vi "Distancias_ejes_convoy_baja_velocidad.vi"(3 "Radios ruedas":dbl[](array[numeric]), 4 "Series_flota1":string[](array[string]), 5 "Ejes_UT":i32[](array[numeric]), 6 "Puntos medios de las ventanas":dbl[][](array[numeric]), 7 "Series_flota":string[](array[string])) -> (0 "Radios_por_ejes":dbl[](array[numeric]), 1 "Distancias_entre_ejes_convoy":dbl[](array[numeric]))   [LabVIEW 2015]
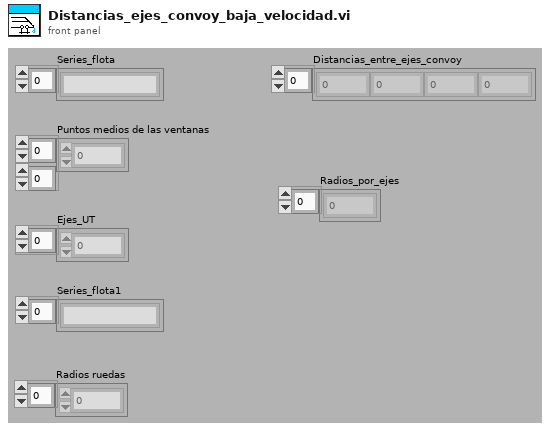
[diagram p1: front panel]
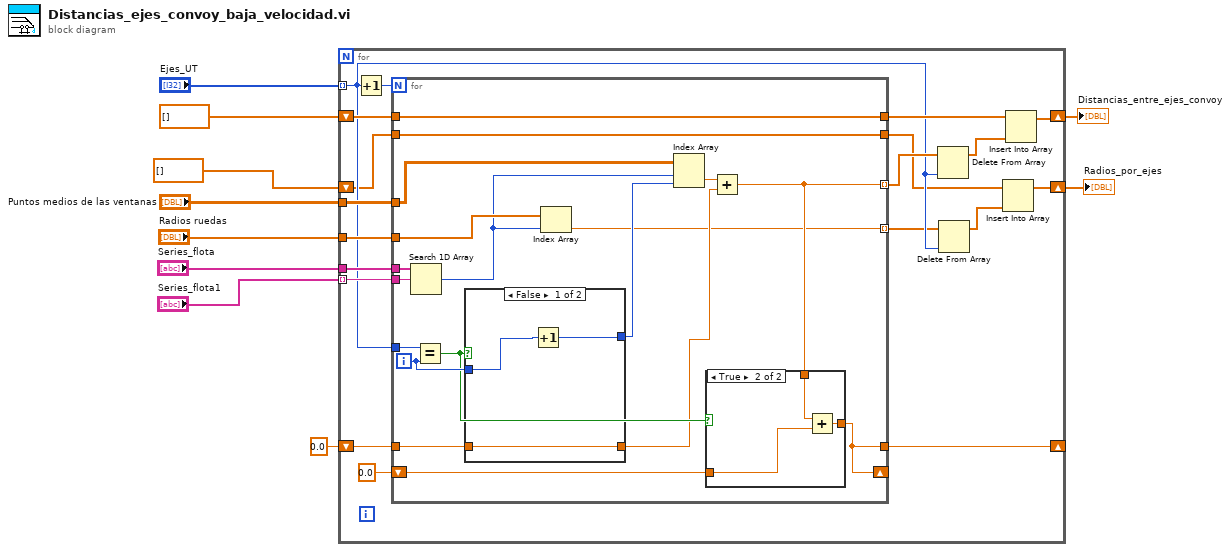
[diagram p0: block diagram]
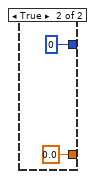
[diagram p3: hidden frame]
diagram:
  n1 = for {
    tunnel: "Puntos medios de las ventanas" -> [w29]
    tunnel: "Ejes_UT" -> [w16] mode=indexing
    tunnel: "Series_flota" -> [w27]
    tunnel: "Series_flota1" -> [w26] mode=indexing
    shift-right: [w23] -> w8
    shift-left: dbl[] [] -> [w25]
    shift-right: [w18] -> _
    shift-left: 0.0 -> [w19]
    tunnel: "Radios ruedas" -> [w17]
    shift-right: [w11] -> w1
    shift-left: dbl[] [] -> [w13]
    n2 = Increment(x=w16) -> (x+1=w28:i32)
    n3 = for {
      N: w28 -> [_]
      tunnel: w29 -> [w42]
      tunnel: w16 -> [w45]
      tunnel: w27 -> [w44]
      tunnel: w26 -> [w43]
      tunnel: [w39] -> w22 mode=indexing
      tunnel: w25 -> [w41]
      tunnel: [w41] -> w24
      shift-right: [w37] -> _
      shift-left: 0.0 -> [w40]
      tunnel: w19 -> [w35]
      tunnel: [w37] -> w18
      tunnel: w17 -> [w33]
      tunnel: [w31] -> w15 mode=indexing
      tunnel: [w30] -> w12
      tunnel: w13 -> [w30]
      i -> [w47]
      n4 = Search 1D Array(1D array=w44, element=w43) -> (index of element=w32:i32)  [unwired: 1 in]
      n5 = Equal?(x=w45, y=w47) -> (x = y?=w38:bool)
      n6 = case shown="False" w38 {
        tunnel: w47 -> [w54 _]
        tunnel: [w53 0] -> w46
        tunnel: w35 -> [w52 _]
        tunnel: [w52 0.0] -> w34
        frame False {
          n7 = Increment(x=w54) -> (x+1=w53:i32)
        }
        frame True {
        }
      }
      n8 = Index Array(array=w33, index=w32) -> (element=w31:dbl)
      n9 = Index Array(array=w42, index (row)=w32, index (col)=w46) -> (element=w36:dbl)
      n10 = Add(x=w36, y=w34) -> (x+y=w39:dbl)
      n11 = case shown="True" w38 {
        tunnel: [w48 w50] -> w37
        tunnel: w39 -> [w48 w51]
        tunnel: w40 -> [_ w49]
        frame False {
        }
        frame True {
          n12 = Add(x=w51, y=w49) -> (x+y=w50:dbl)
        }
      }
    }
    n13 = Delete From Array(array=w22, index=w16) -> (array with subset deleted=w21:dbl[])  [unwired: 1 in, 1 out]
    n14 = Delete From Array(array=w15, index=w16) -> (array with subset deleted=w14:dbl[])  [unwired: 1 in, 1 out]
    n15 = Insert Into Array(array=w12, new element=w14) -> (w11:dbl[])  [unwired: 1 in]
    n16 = Insert Into Array(array=w24, new element=w21) -> (w23:dbl[])  [unwired: 1 in]
  }
  "Distancias_entre_ejes_convoy" <- w8
  "Radios_por_ejes" <- w1
